vi "Get Template LVClass.vi"(10 "LVClass Simple Name":string="QObject.lvclass", 11 "LVLib":refnum<vi>) -> (2 "Object Ref":refnum<vi>, 3 "LVLib Dup":refnum<vi>)   [LabVIEW 2013]
uses:
  <userlib>/ICON Technologies/ICON Maps/lvlib/Map.ctl
  <userlib>/ICON Technologies/ICON Maps/lvlib/_Polymorphic Instances/Map_Insert_Variant.vi
  <userlib>/ICON Technologies/ICON Maps/lvlib/_Polymorphic Instances/Map_Value_Variant.vi
  <userlib>/ICON Technologies/ICON Maps/ICON Maps.lvlib
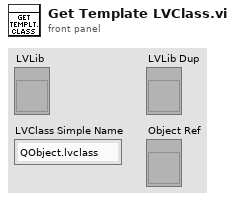
[diagram p1: front panel]
types:
  T1 = typedef "ICON Maps.lvlib/Map.ctl" = variant
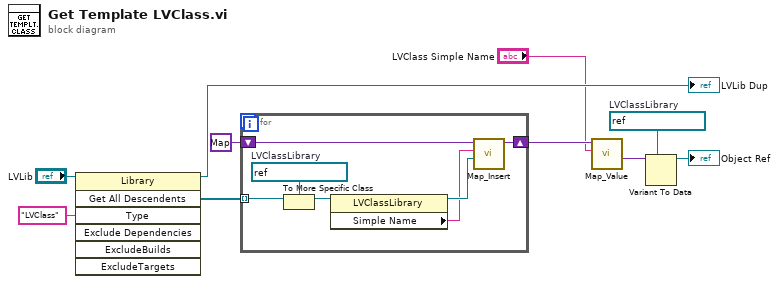
[diagram p0: block diagram]
diagram:
  w3 = refnum<vi> refnum  # LVClassLibrary
  n1 = invoke class="Library" method="Get All Descendents"(reference="LVLib", "Type"="LVClass") -> (reference out=→"LVLib Dup":refnum<vi>, "All Descendents"=w7:refnum<vi>[])  [unwired: 5 in, 5 out]
  n2 = for {
    tunnel: w7 -> [w15] mode=indexing
    shift-right: [w12] -> w5
    shift-left: T1 variant ("Map Out") -> [w13]
    w17 = refnum<vi> refnum  # LVClassLibrary
    n3 = To More Specific Class(target class=w17, reference=w15) -> (specific class reference=w16:refnum<vi>)  [unwired: 1 in, 1 out]
    n4 = property class="LVClassLibrary"(reference=w16) -> (reference out=w14:refnum<vi>, "Simple Name"=w11:string)  [unwired: 1 in, 1 out]
    n5 = call-poly <userlib>:"Map_Insert.vi"("Value"=w14, "Key"=w11, "Map In"=w13) -> ("Map Out"=w12:T1)  [unwired: 8 in]
  }
  n6 = call-poly <userlib>:"Map_Value.vi"("Key"="LVClass Simple Name", "Map In"=w5) -> ("Value"=w2:variant)  [unwired: 8 in, 1 out]
  n7 = Variant To Data(type=w3, Variant=w2) -> (data=→"Object Ref":refnum<vi>)  [unwired: 1 in, 1 out]
